vi "to do.vi"   [LabVIEW 2019]
uses:
  <userlib>/Nanonis Prog Interface/Nanonis Prog Interface.lvlib
  <userlib>/Nanonis Prog Interface/Scan/Grid/GridPatternGet.vi
  <userlib>/Nanonis Prog Interface/Scan/Grid/GridPatternSet.vi
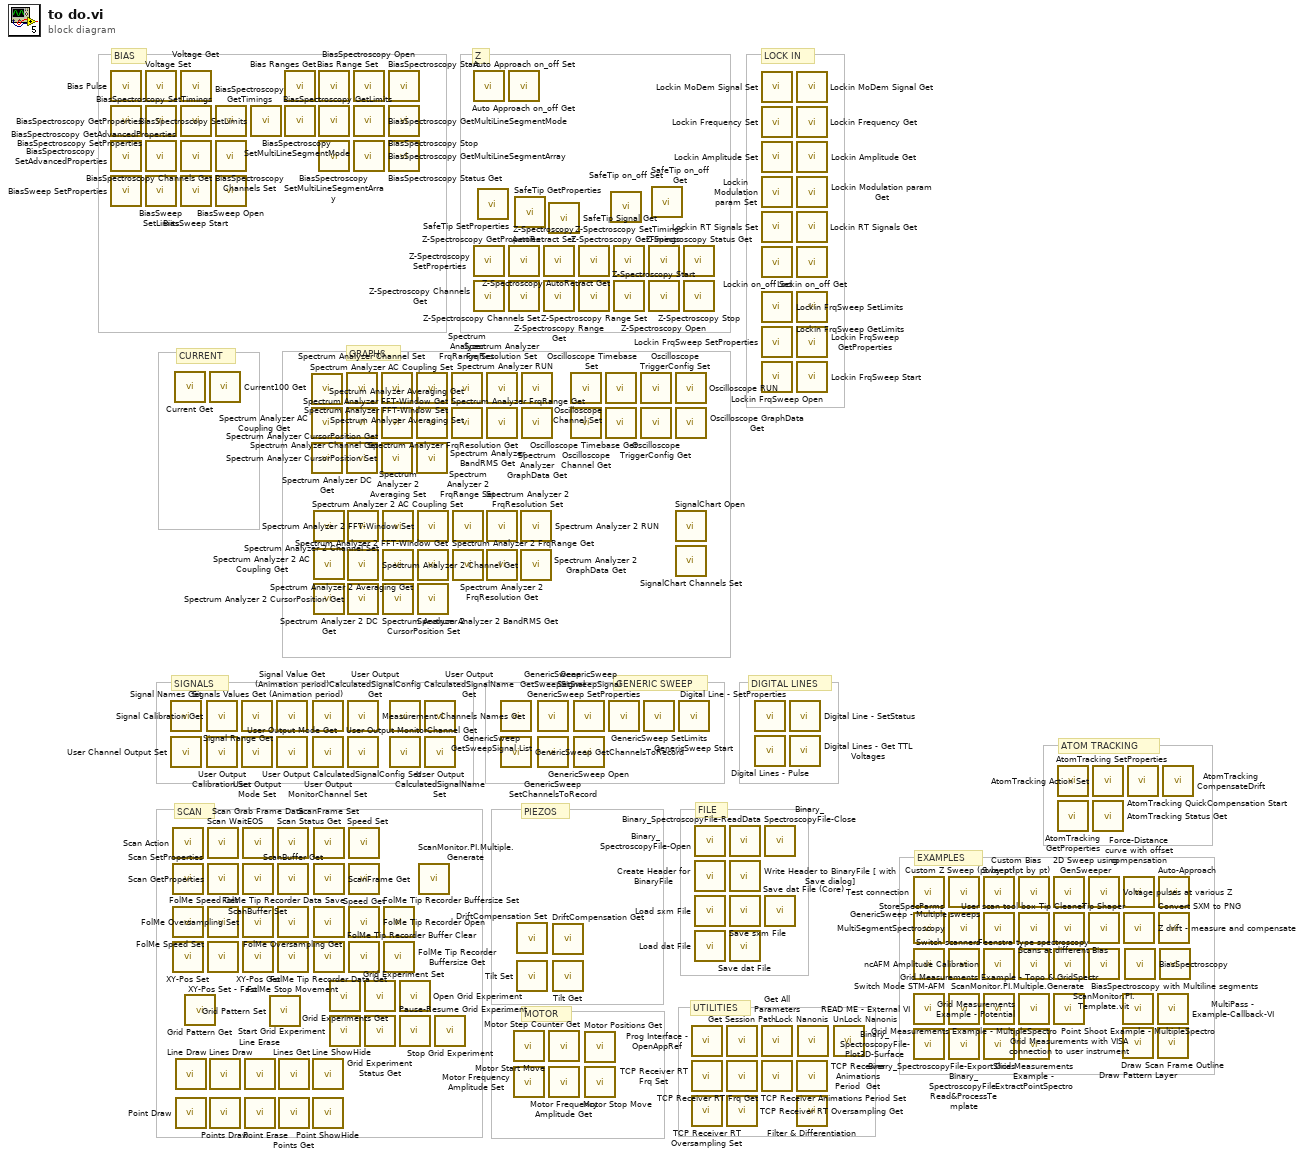
[diagram p0: block diagram]
diagram:
  # "GRAPHS"
  # "ATOM TRACKING"
  # "PIEZOS"
  # "DIGITAL LINES"
  # "FILE"
  # "Z"
  # "UTILITIES"
  # "GENERIC SWEEP"
  # "SIGNALS"
  # "SCAN"
  # "LOCK IN"
  # "EXAMPLES"
  # "CURRENT"
  # "MOTOR"
  # "BIAS"
  n1 = call <userlib>:"Bias Pulse.vi"() -> ()  [unwired: 14 in, 2 out]
  n2 = call <userlib>:"BiasSpectroscopy SetProperties.vi"() -> ()  [unwired: 14 in, 2 out]
  n3 = call <userlib>:"BiasSpectroscopy SetAdvancedProperties.vi"() -> ()  [unwired: 14 in, 2 out]
  n4 = call <userlib>:"BiasSweep SetProperties.vi"() -> ()  [unwired: 14 in, 2 out]
  n5 = call <userlib>:"Voltage Set.vi"() -> ()  [unwired: 10 in, 2 out]
  n6 = call <userlib>:"BiasSpectroscopy GetProperties.vi"() -> ()  [unwired: 8 in, 8 out]
  n7 = call <userlib>:"BiasSpectroscopy GetAdvancedProperties.vi"() -> ()  [unwired: 10 in, 6 out]
  n8 = call <userlib>:"BiasSweep SetLimits.vi"() -> ()  [unwired: 8 in, 2 out]
  n9 = call <userlib>:"Signal Names Get.vi"() -> ()  [unwired: 7 in, 3 out]
  n10 = call <userlib>:"User Channel Output Set.vi"() -> ()  [unwired: 9 in, 2 out]
  n11 = call <userlib>:"Scan Action.vi"() -> ()  [unwired: 9 in, 2 out]
  n12 = call <userlib>:"Scan SetProperties.vi"() -> ()  [unwired: 14 in, 2 out]
  n13 = call <userlib>:"FolMe Speed Set.vi"() -> ()  [unwired: 8 in, 2 out]
  n14 = call <userlib>:"XY-Pos Set.vi"() -> ()  [unwired: 8 in, 2 out]
  n15 = call <userlib>:"Current Get.vi"() -> ()  [unwired: 7 in, 3 out]
  n16 = call <userlib>:"Line Draw.vi"() -> ()  [unwired: 14 in, 2 out]
  n17 = call <userlib>:"Point Draw.vi"() -> ()  [unwired: 14 in, 2 out]
  n18 = call <userlib>:"Voltage Get.vi"() -> ()  [unwired: 9 in, 3 out]
  n19 = call <userlib>:"BiasSpectroscopy SetTimings.vi"() -> ()  [unwired: 14 in, 2 out]
  n20 = call <userlib>:"BiasSpectroscopy Channels Get.vi"() -> ()  [unwired: 9 in, 3 out]
  n21 = call <userlib>:"BiasSweep Start.vi"() -> ()  [unwired: 8 in, 4 out]
  n22 = call-poly <userlib>:"Grid Pattern Get.vi"() -> ()  [unwired: 11 in, 9 out]
  n23 = call <userlib>:"Signal Calibration Get.vi"() -> ()  [unwired: 7 in, 4 out]
  n24 = call <userlib>:"User Output Calibration Set.vi"() -> ()  [unwired: 14 in, 2 out]
  n25 = call <userlib>:"Scan WaitEOS.vi"() -> ()  [unwired: 7 in, 4 out]
  n26 = call <userlib>:"Scan GetProperties.vi"() -> ()  [unwired: 9 in, 7 out]
  n27 = call <userlib>:"FolMe Speed Get.vi"() -> ()  [unwired: 6 in, 4 out]
  n28 = call <userlib>:"XY-Pos Set - Fast.vi"() -> ()  [unwired: 9 in, 2 out]
  n29 = call <userlib>:"Current100 Get.vi"() -> ()  [unwired: 7 in, 3 out]
  n30 = call <userlib>:"Lines Draw.vi"() -> ()  [unwired: 14 in, 2 out]
  n31 = call <userlib>:"Points Draw.vi"() -> ()  [unwired: 14 in, 2 out]
  n32 = call <userlib>:"BiasSpectroscopy GetTimings.vi"() -> ()  [unwired: 11 in, 5 out]
  n33 = call <userlib>:"BiasSpectroscopy Channels Set.vi"() -> ()  [unwired: 10 in, 2 out]
  n34 = call <userlib>:"BiasSweep Open.vi"() -> ()  [unwired: 14 in, 2 out]
  n35 = call <userlib>:"Signal Range Get.vi"() -> ()  [unwired: 7 in, 4 out]
  n36 = call <userlib>:"User Output Mode Set.vi"() -> ()  [unwired: 9 in, 2 out]
  n37 = call <userlib>:"Scan Grab Frame Data.vi"() -> ()  [unwired: 11 in, 5 out]
  n38 = call <userlib>:"ScanBuffer Set.vi"() -> ()  [unwired: 14 in, 2 out]
  n39 = call <userlib>:"FolMe Oversampling Set.vi"() -> ()  [unwired: 8 in, 2 out]
  n40 = call <userlib>:"XY-Pos Get.vi"() -> ()  [unwired: 7 in, 4 out]
  n41 = call <userlib>:"Line Erase.vi"() -> ()  [unwired: 14 in, 2 out]
  n42 = call <userlib>:"Point Erase.vi"() -> ()  [unwired: 14 in, 2 out]
  n43 = call <userlib>:"BiasSpectroscopy SetLimits.vi"() -> ()  [unwired: 8 in, 2 out]
  n44 = call-poly <userlib>:"Grid Pattern Set.vi"() -> ()  [unwired: 18 in, 2 out]
  n45 = call <userlib>:"Signal Value Get (Animation period).vi"() -> ()  [unwired: 8 in, 3 out]
  n46 = call <userlib>:"User Output Mode Get.vi"() -> ()  [unwired: 7 in, 3 out]
  n47 = call <userlib>:"Scan Status Get.vi"() -> ()  [unwired: 8 in, 3 out]
  n48 = call <userlib>:"ScanBuffer Get.vi"() -> ()  [unwired: 11 in, 5 out]
  n49 = call <userlib>:"FolMe Oversampling Get.vi"() -> ()  [unwired: 6 in, 4 out]
  n50 = call <userlib>:"FolMe Stop Movement.vi"() -> ()  [unwired: 8 in, 2 out]
  n51 = call <userlib>:"Lines Get.vi"() -> ()  [unwired: 13 in, 3 out]
  n52 = call <userlib>:"Points Get.vi"() -> ()  [unwired: 13 in, 3 out]
  n53 = call <userlib>:"Bias Ranges Get.vi"() -> ()  [unwired: 8 in, 4 out]
  n54 = call <userlib>:"BiasSpectroscopy GetLimits.vi"() -> ()  [unwired: 6 in, 4 out]
  n55 = call <userlib>:"Spectrum Analyzer AC Coupling Set.vi"() -> ()  [unwired: 10 in, 2 out]
  n56 = call <userlib>:"Spectrum Analyzer AC Coupling Get.vi"() -> ()  [unwired: 9 in, 3 out]
  n57 = call <userlib>:"Spectrum Analyzer DC Get.vi"() -> ()  [unwired: 9 in, 3 out]
  n58 = call <userlib>:"Signals Values Get (Animation period).vi"() -> ()  [unwired: 8 in, 3 out]
  n59 = call <userlib>:"User Output MonitorChannel Set.vi"() -> ()  [unwired: 9 in, 2 out]
  n60 = call <userlib>:"Line ShowHide.vi"() -> ()  [unwired: 14 in, 2 out]
  n61 = call <userlib>:"Point ShowHide.vi"() -> ()  [unwired: 14 in, 2 out]
  n62 = call <userlib>:"Spectrum Analyzer 2 AC Coupling Set.vi"() -> ()  [unwired: 10 in, 2 out]
  n63 = call <userlib>:"Spectrum Analyzer 2 AC Coupling Get.vi"() -> ()  [unwired: 9 in, 3 out]
  n64 = call <userlib>:"Spectrum Analyzer 2 DC Get.vi"() -> ()  [unwired: 9 in, 3 out]
  n65 = call <userlib>:"ScanFrame Set.vi"() -> ()  [unwired: 14 in, 2 out]
  n66 = call <userlib>:"ScanFrame Get.vi"() -> ()  [unwired: 11 in, 5 out]
  n67 = call <userlib>:"FolMe Tip Recorder Data Save.vi"() -> ()  [unwired: 10 in, 2 out]
  n68 = call <userlib>:"FolMe Tip Recorder Data Get.vi"() -> ()  [unwired: 8 in, 4 out]
  n69 = call <userlib>:"Bias Range Set.vi"() -> ()  [unwired: 10 in, 2 out]
  n70 = call <userlib>:"BiasSpectroscopy SetMultiLineSegmentMode.vi"() -> ()  [unwired: 8 in, 2 out]
  n71 = call <userlib>:"BiasSpectroscopy SetMultiLineSegmentArray.vi"() -> ()  [unwired: 8 in, 2 out]
  n72 = call <userlib>:"Grid Experiments Get.vi"() -> ()  [unwired: 13 in, 7 out]
  n73 = call <userlib>:"Start Grid Experiment.vi"() -> ()  [unwired: 18 in, 2 out]
  n74 = call <userlib>:"Spectrum Analyzer Channel Set.vi"() -> ()  [unwired: 10 in, 2 out]
  n75 = call <userlib>:"Spectrum Analyzer Channel Get.vi"() -> ()  [unwired: 9 in, 3 out]
  n76 = call <userlib>:"Spectrum Analyzer CursorPosition Get.vi"() -> ()  [unwired: 11 in, 5 out]
  n77 = call <userlib>:"Spectrum Analyzer 2 Channel Set.vi"() -> ()  [unwired: 10 in, 2 out]
  n78 = call <userlib>:"Spectrum Analyzer 2 Channel Get.vi"() -> ()  [unwired: 9 in, 3 out]
  n79 = call <userlib>:"Spectrum Analyzer 2 CursorPosition Get.vi"() -> ()  [unwired: 11 in, 5 out]
  n80 = call <userlib>:"Measurement Channels Names Get.vi"() -> ()  [unwired: 9 in, 3 out]
  n81 = call <userlib>:"User Output MonitorChannel Get.vi"() -> ()  [unwired: 8 in, 3 out]
  n82 = call <userlib>:"Speed Set.vi"() -> ()  [unwired: 14 in, 2 out]
  n83 = call <userlib>:"Speed Get.vi"() -> ()  [unwired: 10 in, 6 out]
  n84 = call <userlib>:"FolMe Tip Recorder Open.vi"() -> ()  [unwired: 8 in, 2 out]
  n85 = call <userlib>:"FolMe Tip Recorder Buffer Clear.vi"() -> ()  [unwired: 8 in, 2 out]
  n86 = call <userlib>:"BiasSpectroscopy Open.vi"() -> ()  [unwired: 14 in, 2 out]
  n87 = call <userlib>:"BiasSpectroscopy GetMultiLineSegmentMode.vi"() -> ()  [unwired: 7 in, 3 out]
  n88 = call <userlib>:"BiasSpectroscopy GetMultiLineSegmentArray.vi"() -> ()  [unwired: 7 in, 3 out]
  n89 = call <userlib>:"Grid Experiment Set.vi"() -> ()  [unwired: 18 in, 2 out]
  n90 = call <userlib>:"Grid Experiment Status Get.vi"() -> ()  [unwired: 9 in, 3 out]
  n91 = call <userlib>:"Spectrum Analyzer Averaging Set.vi"() -> ()  [unwired: 10 in, 2 out]
  n92 = call <userlib>:"Spectrum Analyzer Averaging Get.vi"() -> ()  [unwired: 9 in, 3 out]
  n93 = call <userlib>:"Spectrum Analyzer CursorPosition Set.vi"() -> ()  [unwired: 14 in, 2 out]
  n94 = call <userlib>:"Spectrum Analyzer 2 Averaging Set.vi"() -> ()  [unwired: 10 in, 2 out]
  n95 = call <userlib>:"Spectrum Analyzer 2 Averaging Get.vi"() -> ()  [unwired: 9 in, 3 out]
  n96 = call <userlib>:"Spectrum Analyzer 2 CursorPosition Set.vi"() -> ()  [unwired: 14 in, 2 out]
  n97 = call <userlib>:"FolMe Tip Recorder Buffersize Set.vi"() -> ()  [unwired: 8 in, 2 out]
  n98 = call <userlib>:"FolMe Tip Recorder Buffersize Get.vi"() -> ()  [unwired: 7 in, 3 out]
  n99 = call <userlib>:"BiasSpectroscopy Start.vi"() -> ()  [unwired: 11 in, 5 out]
  n100 = call <userlib>:"BiasSpectroscopy Stop.vi"() -> ()  [unwired: 14 in, 2 out]
  n101 = call <userlib>:"BiasSpectroscopy Status Get.vi"() -> ()  [unwired: 7 in, 3 out]
  n102 = call <userlib>:"User Output CalculatedSignalConfig Get.vi"() -> ()  [unwired: 8 in, 3 out]
  n103 = call <userlib>:"User Output CalculatedSignalConfig Set.vi"() -> ()  [unwired: 9 in, 2 out]
  n104 = call <userlib>:"Open Grid Experiment.vi"() -> ()  [unwired: 18 in, 2 out]
  n105 = call <userlib>:"Pause-Resume Grid Experiment.vi"() -> ()  [unwired: 18 in, 2 out]
  n106 = call <userlib>:"Spectrum Analyzer FFT-Window Set.vi"() -> ()  [unwired: 10 in, 2 out]
  n107 = call <userlib>:"Spectrum Analyzer FFT-Window Get.vi"() -> ()  [unwired: 9 in, 3 out]
  n108 = call <userlib>:"Spectrum Analyzer BandRMS Get.vi"() -> ()  [unwired: 8 in, 4 out]
  n109 = call <userlib>:"Spectrum Analyzer 2 FFT-Window Set.vi"() -> ()  [unwired: 10 in, 2 out]
  n110 = call <userlib>:"Spectrum Analyzer 2 FFT-Window Get.vi"() -> ()  [unwired: 9 in, 3 out]
  n111 = call <userlib>:"Spectrum Analyzer 2 BandRMS Get.vi"() -> ()  [unwired: 8 in, 4 out]
  n112 = call <userlib>:"ScanMonitor.PI.Multiple.Generate.vi"() -> ()  [unwired: 1 in]
  n113 = call <userlib>:"User Output CalculatedSignalName Get.vi"() -> ()  [unwired: 8 in, 3 out]
  n114 = call <userlib>:"User Output CalculatedSignalName Set.vi"() -> ()  [unwired: 9 in, 2 out]
  n115 = call <userlib>:"Stop Grid Experiment.vi"() -> ()  [unwired: 18 in, 2 out]
  n116 = call <userlib>:"Spectrum Analyzer FrqRange Set.vi"() -> ()  [unwired: 10 in, 2 out]
  n117 = call <userlib>:"Spectrum Analyzer FrqRange Get.vi"() -> ()  [unwired: 8 in, 4 out]
  n118 = call <userlib>:"Spectrum Analyzer 2 FrqRange Set.vi"() -> ()  [unwired: 10 in, 2 out]
  n119 = call <userlib>:"Spectrum Analyzer 2 FrqRange Get.vi"() -> ()  [unwired: 8 in, 4 out]
  n120 = call <userlib>:"Auto Approach on_off Set.vi"() -> ()  [unwired: 8 in, 2 out]
  n121 = call <userlib>:"Z-Spectroscopy SetProperties.vi"() -> ()  [unwired: 14 in, 2 out]
  n122 = call <userlib>:"Z-Spectroscopy Channels Get.vi"() -> ()  [unwired: 9 in, 3 out]
  n123 = call <userlib>:"SafeTip SetProperties.vi"() -> ()  [unwired: 14 in, 2 out]
  n124 = call <userlib>:"Spectrum Analyzer FrqResolution Set.vi"() -> ()  [unwired: 10 in, 2 out]
  n125 = call <userlib>:"Spectrum Analyzer FrqResolution Get.vi"() -> ()  [unwired: 8 in, 4 out]
  n126 = call <userlib>:"Spectrum Analyzer 2 FrqResolution Set.vi"() -> ()  [unwired: 10 in, 2 out]
  n127 = call <userlib>:"Spectrum Analyzer 2 FrqResolution Get.vi"() -> ()  [unwired: 8 in, 4 out]
  n128 = call <userlib>:"GenericSweep GetSweepSignal List.vi"() -> ()  [unwired: 9 in, 3 out]
  n129 = call <userlib>:"GenericSweep GetChannelsToRecord.vi"() -> ()  [unwired: 8 in, 4 out]
  n130 = call <userlib>:"Auto Approach on_off Get.vi"() -> ()  [unwired: 7 in, 3 out]
  n131 = call <userlib>:"Z-Spectroscopy GetProperties.vi"() -> ()  [unwired: 8 in, 8 out]
  n132 = call <userlib>:"Z-Spectroscopy Channels Set.vi"() -> ()  [unwired: 10 in, 2 out]
  n133 = call <userlib>:"Motor Start Move.vi"() -> ()  [unwired: 9 in, 2 out]
  n134 = call <userlib>:"Motor Frequency Amplitude Set.vi"() -> ()  [unwired: 10 in, 2 out]
  n135 = call <userlib>:"SafeTip GetProperties.vi"() -> ()  [unwired: 11 in, 5 out]
  n136 = call <userlib>:"DriftCompensation Set.vi"() -> ()  [unwired: 14 in, 2 out]
  n137 = call <userlib>:"Tilt Set.vi"() -> ()  [unwired: 10 in, 2 out]
  n138 = call <userlib>:"Spectrum Analyzer 2 RUN.vi"() -> ()  [unwired: 10 in, 2 out]
  n139 = call <userlib>:"Spectrum Analyzer 2 GraphData Get.vi"() -> ()  [unwired: 9 in, 3 out]
  n140 = call <userlib>:"Spectrum Analyzer RUN.vi"() -> ()  [unwired: 10 in, 2 out]
  n141 = call <userlib>:"Spectrum Analyzer GraphData Get.vi"() -> ()  [unwired: 9 in, 3 out]
  n142 = call <userlib>:"GenericSweep GetSweepSignal.vi"() -> ()  [unwired: 8 in, 4 out]
  n143 = call <userlib>:"GenericSweep SetChannelsToRecord.vi"() -> ()  [unwired: 10 in, 2 out]
  n144 = call <userlib>:"Z-Spectroscopy AutoRetract Set.vi"() -> ()  [unwired: 10 in, 2 out]
  n145 = call <userlib>:"Z-Spectroscopy Range Get.vi"() -> ()  [unwired: 7 in, 4 out]
  n146 = call <userlib>:"SafeTip Signal Get.vi"() -> ()  [unwired: 9 in, 3 out]
  n147 = call <userlib>:"Motor Step Counter Get.vi"() -> ()  [unwired: 11 in, 5 out]
  n148 = call <userlib>:"Motor Frequency Amplitude Get.vi"() -> ()  [unwired: 8 in, 4 out]
  n149 = call <userlib>:"DriftCompensation Get.vi"() -> ()  [unwired: 11 in, 5 out]
  n150 = call <userlib>:"Tilt Get.vi"() -> ()  [unwired: 8 in, 4 out]
  n151 = call <userlib>:"Oscilloscope Channel Set.vi"() -> ()  [unwired: 10 in, 2 out]
  n152 = call <userlib>:"Oscilloscope Channel Get.vi"() -> ()  [unwired: 9 in, 3 out]
  n153 = call <userlib>:"GenericSweep SetSweepSignal.vi"() -> ()  [unwired: 10 in, 2 out]
  n154 = call <userlib>:"GenericSweep Open.vi"() -> ()  [unwired: 14 in, 2 out]
  n155 = call <userlib>:"Z-Spectroscopy AutoRetract Get.vi"() -> ()  [unwired: 6 in, 6 out]
  n156 = call <userlib>:"Z-Spectroscopy Range Set.vi"() -> ()  [unwired: 9 in, 2 out]
  n157 = call <userlib>:"Motor Positions Get.vi"() -> ()  [unwired: 11 in, 5 out]
  n158 = call <userlib>:"Motor Stop Move.vi"() -> ()  [unwired: 10 in, 2 out]
  n159 = call <userlib>:"Oscilloscope Timebase Set.vi"() -> ()  [unwired: 10 in, 2 out]
  n160 = call <userlib>:"Oscilloscope Timebase Get.vi"() -> ()  [unwired: 8 in, 4 out]
  n161 = call <userlib>:"GenericSweep SetProperties.vi"() -> ()  [unwired: 14 in, 2 out]
  n162 = call <userlib>:"SafeTip on_off Set.vi"() -> ()  [unwired: 10 in, 2 out]
  n163 = call <userlib>:"Z-Spectroscopy SetTimings.vi"() -> ()  [unwired: 14 in, 2 out]
  n164 = call <userlib>:"Z-Spectroscopy Start.vi"() -> ()  [unwired: 11 in, 5 out]
  n165 = call <userlib>:"Oscilloscope TriggerConfig Set.vi"() -> ()  [unwired: 10 in, 2 out]
  n166 = call <userlib>:"Oscilloscope TriggerConfig Get.vi"() -> ()  [unwired: 8 in, 4 out]
  n167 = call <userlib>:"GenericSweep SetLimits.vi"() -> ()  [unwired: 8 in, 2 out]
  n168 = call <userlib>:"Z-Spectroscopy GetTimings.vi"() -> ()  [unwired: 11 in, 5 out]
  n169 = call <userlib>:"Z-Spectroscopy Open.vi"() -> ()  [unwired: 14 in, 2 out]
  n170 = call <userlib>:"SafeTip on_off Get.vi"() -> ()  [unwired: 9 in, 3 out]
  n171 = call <userlib>:"Oscilloscope RUN.vi"() -> ()  [unwired: 10 in, 2 out]
  n172 = call <userlib>:"Oscilloscope GraphData Get.vi"() -> ()  [unwired: 9 in, 3 out]
  n173 = call <userlib>:"SignalChart Open.vi"() -> ()  [unwired: 10 in, 2 out]
  n174 = call <userlib>:"SignalChart Channels Set.vi"() -> ()  [unwired: 10 in, 2 out]
  n175 = call <userlib>:"GenericSweep Start.vi"() -> ()  [unwired: 12 in, 4 out]
  n176 = call <userlib>:"Z-Spectroscopy Status Get.vi"() -> ()  [unwired: 7 in, 3 out]
  n177 = call <userlib>:"Z-Spectroscopy Stop.vi"() -> ()  [unwired: 14 in, 2 out]
  n178 = call <userlib>:"Prog Interface - OpenAppRef.vi"() -> ()  [unwired: 6 in, 2 out]
  n179 = call <userlib>:"TCP Receiver RT Frq Set.vi"() -> ()  [unwired: 10 in, 2 out]
  n180 = call <userlib>:"TCP Receiver RT Oversampling Set.vi"() -> ()  [unwired: 10 in, 2 out]
  n181 = call <userlib>:"Binary_SpectroscopyFile-Open.vi"() -> ()  [unwired: 7 in, 5 out]
  n182 = call <userlib>:"Create Header for BinaryFile.vi"() -> ()  [unwired: 11 in, 1 out]
  n183 = call <userlib>:"Load sxm File.vi"() -> ()  [unwired: 6 in, 6 out]
  n184 = call <userlib>:"Load dat File.vi"() -> ()  [unwired: 8 in, 4 out]
  n185 = call <userlib>:"Get Session Path.vi"() -> ()  [unwired: 9 in, 3 out]
  n186 = call <userlib>:"TCP Receiver RT Frq Get.vi"() -> ()  [unwired: 9 in, 3 out]
  n187 = call <userlib>:"TCP Receiver RT Oversampling Get.vi"() -> ()  [unwired: 9 in, 3 out]
  n188 = call <userlib>:"Binary_SpectroscopyFile-ReadData.vi"() -> ()  [unwired: 8 in, 4 out]
  n189 = call <userlib>:"Write Header to BinaryFile [ with Save dialog].vi"() -> ()  [unwired: 8 in, 4 out]
  n190 = call <userlib>:"Save sxm File.vi"() -> ()  [unwired: 9 in, 3 out]
  n191 = call <userlib>:"Save dat File.vi"() -> ()  [unwired: 12 in, 4 out]
  n192 = call <userlib>:"Digital Line - SetProperties.vi"() -> ()  [unwired: 9 in, 3 out]
  n193 = call <userlib>:"Digital Lines - Pulse.vi"() -> ()  [unwired: 13 in, 3 out]
  n194 = call <userlib>:"Lockin MoDem Signal Set.vi"() -> ()  [unwired: 10 in, 2 out]
  n195 = call <userlib>:"Lockin Frequency Set.vi"() -> ()  [unwired: 10 in, 2 out]
  n196 = call <userlib>:"Lockin Amplitude Set.vi"() -> ()  [unwired: 10 in, 2 out]
  n197 = call <userlib>:"Lockin Modulation param Set.vi"() -> ()  [unwired: 14 in, 2 out]
  n198 = call <userlib>:"Lockin RT Signals Set.vi"() -> ()  [unwired: 10 in, 2 out]
  n199 = call <userlib>:"Lockin on_off Set.vi"() -> ()  [unwired: 10 in, 2 out]
  n200 = call <userlib>:"Lockin FrqSweep SetLimits.vi"() -> ()  [unwired: 10 in, 2 out]
  n201 = call <userlib>:"Lockin FrqSweep SetProperties.vi"() -> ()  [unwired: 14 in, 2 out]
  n202 = call <userlib>:"Lockin FrqSweep Open.vi"() -> ()  [unwired: 10 in, 2 out]
  n203 = call <userlib>:"Get All Parameters.vi"() -> ()  [unwired: 9 in, 3 out]
  n204 = call <userlib>:"TCP Receiver Animations Period Set.vi"() -> ()  [unwired: 10 in, 2 out]
  n205 = call <userlib>:"Binary_SpectroscopyFile-Close.vi"() -> ()  [unwired: 11 in, 1 out]
  n206 = call <userlib>:"Save dat File (Core).vi"() -> ()  [unwired: 14 in, 2 out]
  n207 = call <userlib>:"Digital Line - SetStatus.vi"() -> ()  [unwired: 9 in, 3 out]
  n208 = call <userlib>:"Digital Lines - Get TTL Voltages.vi"() -> ()  [unwired: 8 in, 4 out]
  n209 = call <userlib>:"Lockin MoDem Signal Get.vi"() -> ()  [unwired: 8 in, 4 out]
  n210 = call <userlib>:"Lockin Frequency Get.vi"() -> ()  [unwired: 9 in, 3 out]
  n211 = call <userlib>:"Lockin Amplitude Get.vi"() -> ()  [unwired: 9 in, 3 out]
  n212 = call <userlib>:"Lockin Modulation param Get.vi"() -> ()  [unwired: 11 in, 5 out]
  n213 = call <userlib>:"Lockin RT Signals Get.vi"() -> ()  [unwired: 8 in, 4 out]
  n214 = call <userlib>:"Lockin on_off Get.vi"() -> ()  [unwired: 9 in, 3 out]
  n215 = call <userlib>:"Lockin FrqSweep GetLimits.vi"() -> ()  [unwired: 8 in, 4 out]
  n216 = call <userlib>:"Lockin FrqSweep GetProperties.vi"() -> ()  [unwired: 10 in, 6 out]
  n217 = call <userlib>:"Lockin FrqSweep Start.vi"() -> ()  [unwired: 8 in, 4 out]
  n218 = call <userlib>:"TCP Receiver Animations Period  Get.vi"() -> ()  [unwired: 9 in, 3 out]
  n219 = call <userlib>:"Filter & Differentiation.vi"() -> ()  [unwired: 9 in, 3 out]
  n220 = call <userlib>:"Lock Nanonis.vi"() -> ()  [unwired: 10 in, 2 out]
  n221 = call <userlib>:"UnLock Nanonis.vi"() -> ()  [unwired: 10 in, 2 out]
  n222 = call <userlib>:"Test connection.vi"() -> ()  [unwired: 1 in]
  n223 = call <userlib>:"StoreSpecParms.vi"() -> ()  [unwired: 1 in]
  n224 = call <userlib>:"Switch Mode STM-AFM.vi"() -> ()  [unwired: 1 in]
  n225 = call <userlib>:"READ ME - External VI.vi"() -> ()  [unwired: 1 in]
  n226 = call <userlib>:"Binary_SpectroscopyFile-Plot3D-Surface.vi"() -> ()  [unwired: 12 in]
  n227 = call <userlib>:"GenericSweep - Multiple sweeps.vi"() -> ()  [unwired: 1 in]
  n228 = call <userlib>:"MultiSegmentSpectroscopy.vi"() -> ()  [unwired: 1 in]
  n229 = call <userlib>:"Switch scanners.vi"() -> ()  [unwired: 1 in]
  n230 = call <userlib>:"Grid Measurements Example - MultipleSpectro.vi"() -> ()  [unwired: 11 in, 1 out]
  n231 = call <userlib>:"Binary_SpectroscopyFile-Read&ProcessTemplate.vi"() -> ()  [unwired: 1 in]
  n232 = call <userlib>:"Custom Z Sweep (pt by pt).vi"() -> ()  [unwired: 1 in]
  n233 = call <userlib>:"User scan tool box.vi"() -> ()  [unwired: 1 in]
  n234 = call <userlib>:"ncAFM Amplitude Calibration.vi"() -> ()  [unwired: 1 in]
  n235 = call <userlib>:"Grid Measurements Example - Topo & GridSpectr.vi"() -> ()  [unwired: 11 in, 1 out]
  n236 = call <userlib>:"Binary_SpectroscopyFile-ExportSlices.vi"() -> ()  [unwired: 1 in]
  n237 = call <userlib>:"Custom Bias Sweep (pt by pt).vi"() -> ()  [unwired: 1 in]
  n238 = call <userlib>:"Scans at different Bias.vi"() -> ()  [unwired: 1 in]
  n239 = call <userlib>:"Feenstra type spectroscopy.vi"() -> ()  [unwired: 1 in]
  n240 = call <userlib>:"Grid Measurements Example - Potential.vi"() -> ()  [unwired: 11 in, 1 out]
  n241 = call <userlib>:"Grid Measurements Example - ExtractPointSpectro.vi"() -> ()  [unwired: 9 in, 3 out]
  n242 = call <userlib>:"2D Sweep using GenSweeper.vi"() -> ()  [unwired: 1 in]
  n243 = call <userlib>:"Tip Cleaner.vi"() -> ()  [unwired: 1 in]
  n244 = call <userlib>:"ScanMonitor.PI.Multiple.Generate.vi"() -> ()  [unwired: 1 in]
  n245 = call <userlib>:"Grid Measurements with VISA connection to user instrument.vi"() -> ()  [unwired: 11 in, 1 out]
  n246 = call <userlib>:"AtomTracking SetProperties.vi"() -> ()  [unwired: 14 in, 2 out]
  n247 = call <userlib>:"AtomTracking GetProperties.vi"() -> ()  [unwired: 9 in, 7 out]
  n248 = call <userlib>:"Voltage pulses at various Z.vi"() -> ()  [unwired: 1 in]
  n249 = call <userlib>:"Tip Shaper.vi"() -> ()  [unwired: 1 in]
  n250 = call <userlib>:"ScanMonitor.PI.Template.vit"() -> ()  [unwired: 12 in]
  n251 = call <userlib>:"AtomTracking Action Set.vi"() -> ()  [unwired: 10 in, 2 out]
  n252 = call <userlib>:"AtomTracking Status Get.vi"() -> ()  [unwired: 9 in, 3 out]
  n253 = call <userlib>:"Point Shoot Example - MultipleSpectro.vi"() -> ()  [unwired: 11 in, 1 out]
  n254 = call <userlib>:"Draw Pattern Layer.vi"() -> ()  [unwired: 1 in]
  n255 = call <userlib>:"Force-Distance curve with offset compensation.vi"() -> ()  [unwired: 1 in]
  n256 = call <userlib>:"Z drift - measure and compensate.vi"() -> ()  [unwired: 1 in]
  n257 = call <userlib>:"BiasSpectroscopy.vi"() -> ()  [unwired: 1 in]
  n258 = call <userlib>:"AtomTracking QuickCompensation Start.vi"() -> ()  [unwired: 10 in, 2 out]
  n259 = call <userlib>:"MultiPass - Example-Callback-VI.vi"() -> ()  [unwired: 11 in, 1 out]
  n260 = call <userlib>:"Draw Scan Frame Outline.vi"() -> ()  [unwired: 1 in]
  n261 = call <userlib>:"Auto-Approach.vi"() -> ()  [unwired: 1 in]
  n262 = call <userlib>:"Convert SXM to PNG.vi"() -> ()  [unwired: 1 in]
  n263 = call <userlib>:"BiasSpectroscopy with Multiline segments.vi"() -> ()  [unwired: 1 in]
  n264 = call <userlib>:"AtomTracking CompensateDrift.vi"() -> ()  [unwired: 10 in, 2 out]
